vi "GetParam.vi"(8 "error in (no error)":errorcluster caption="entrée d'erreur (pas d'erreur)", 11 "TimeSeriesSplit.lvclass":refnum<class "TimeSeriesSplit.lvclass">) -> (0 "error out":errorcluster caption="sortie d'erreur", 2 "TimeSeriesSplit":cluster{"n_splits":i32, "max_train_size":string}={"n_splits"=5, "max_train_size"="None"}, 3 "TimeSeriesSplit.lvclass":refnum<class "TimeSeriesSplit.lvclass">)   [LabVIEW 2020, in "TimeSeriesSplit.lvclass"]
doc: "Get Parameters"
uses:
  TimeSeriesSplit.lvclass
  TimeSeriesSplit.lvclass/TimeSeriesSplit.ctl
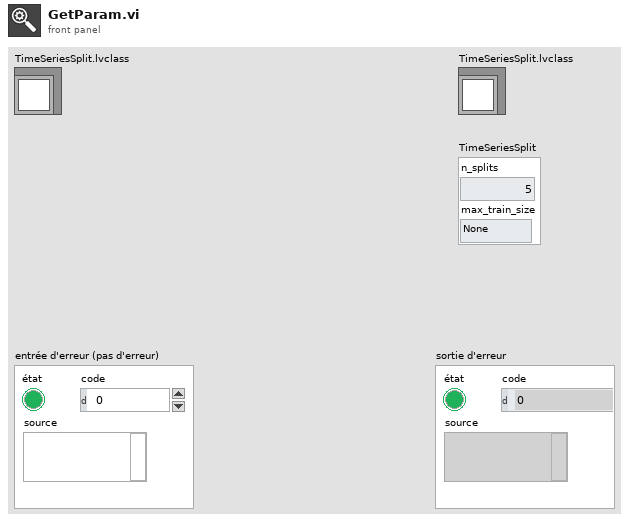
[diagram p1: front panel]
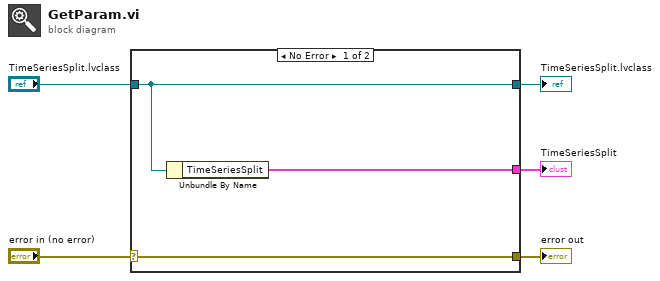
[diagram p0: block diagram]
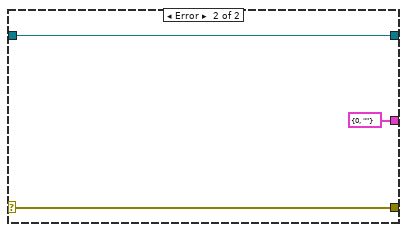
[diagram p2: hidden frame]
diagram:
  n1 = case shown="No Error" "error in (no error)" {
    selector: "error in (no error)" -> [w8 w10]
    tunnel: [w8 w10] -> w4
    tunnel: [w7 w11] -> w2
    tunnel: "TimeSeriesSplit.lvclass" -> [w7 w11]
    tunnel: [w6 cluster{"n_splits":i32, "max_train_size":string} {"n_splits"=0, "max_train_size"=""} ("TimeSeriesSplit")] -> w1
    frame No Error {
      n2 = Unbundle By Name(w7) -> ("TimeSeriesSplit"=w6:cluster{"n_splits":i32, "max_train_size":string})
    }
    frame Error {
    }
  }
  "error out" <- w4
  "TimeSeriesSplit.lvclass" <- w2
  "TimeSeriesSplit" <- w1
